vi "Concatenate Strings If not Empty_csm.vi"(3 "String":string, 4 "seperator(:)":string=":", 5 "prefix":string) -> (1 "result":string)   [LabVIEW 2017, in "API String Arguments Support.lvlib"]
doc: "Concatenate string with <b>separator</b> if two strings are not empty. Otherwise, return raw values without <b>separator</b>. The default value of <b>separator</b> is colon separator(<b>:</b>)."
uses:
  API String Arguments Support.lvlib
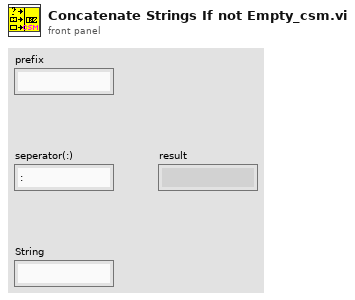
[diagram p1: front panel]
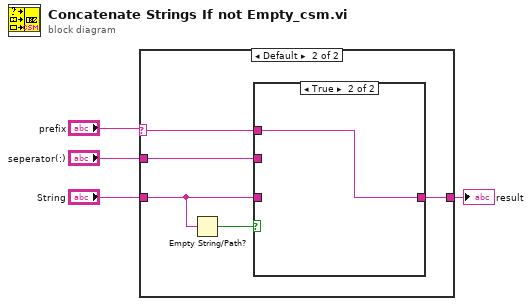
[diagram p0: block diagram]
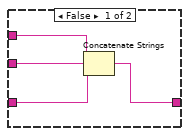
[diagram p3: hidden frame]
diagram:
  n1 = case shown="Default" "prefix" {
    selector: "prefix" -> [_ w9]
    tunnel: "seperator(:)" -> [_ w10]
    tunnel: "String" -> [w5 w7]
    tunnel: [w5 w8] -> w1
    frame "" {
    }
    frame Default {
      n2 = Empty String/Path?(string/path=w7) -> (empty?=w6:bool)
      n3 = case shown="True" w6 {
        tunnel: w10 -> [w14 _]
        tunnel: w9 -> [w13 w15]
        tunnel: [w12 w15] -> w8
        tunnel: w7 -> [w11 _]
        frame False {
          n4 = Concatenate Strings(w13, w14, w11) -> (w12:string)
        }
        frame True {
        }
      }
    }
  }
  "result" <- w1
